vi "Message-Enqueuer References Control Name.vi"() -> (0 "Message Enqueuers Reference Control Name":string="Message-Enqueuer References.ctl")   [LabVIEW 2018, in "Scripting.lvlib"]
uses:
  Scripting.lvlib
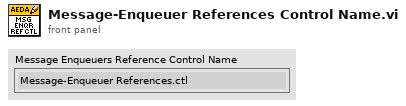
[diagram p1: front panel]
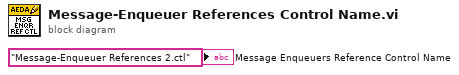
[diagram p0: block diagram]
diagram:
  "Message Enqueuers Reference Control Name" <- "Message-Enqueuer References 2.ctl"
